vi "SerialPort.Function_Config Com Port.vi"(5 "Timeout(ms)":i32=1000, 7 "Module Name":string="Serial Port", 8 "error in":errorcluster, 9 "Port Timeout ms (3000)":u32=3000, 10 "Config":T1={"Baud Rate (115200)"=115200, "Data Bits (8)"=8, "Parity (0:none)"=enum."None", "Stop Bits (10: 1 bit)"=10, "Flow Control (0:none)"=enum."None", "Enable Term Char (T)"=TRUE, "Term Char(0xA = '\\n' = LF) "=10} {"Term Char(0xA = '\\n' = LF)" format="%.0x"; "Stop Bits (10: 1 bit)" items=["1.0"=10, "1.5"=15, "2.0"=20]; "Data Bits (8)" min=5 max=8 step=1}, 11 "Q In":refnum<queue>) -> (0 "error out":errorcluster)   [LabVIEW 2018]
uses:
  <vilib>/KATE/Queues/Q.Element.ctl
  Controls/SeroalPort.Config Settings.ctl
  <vilib>/KATE/Queues/Queue Utils.lvlib
panel:
  # "Serial Port Config"
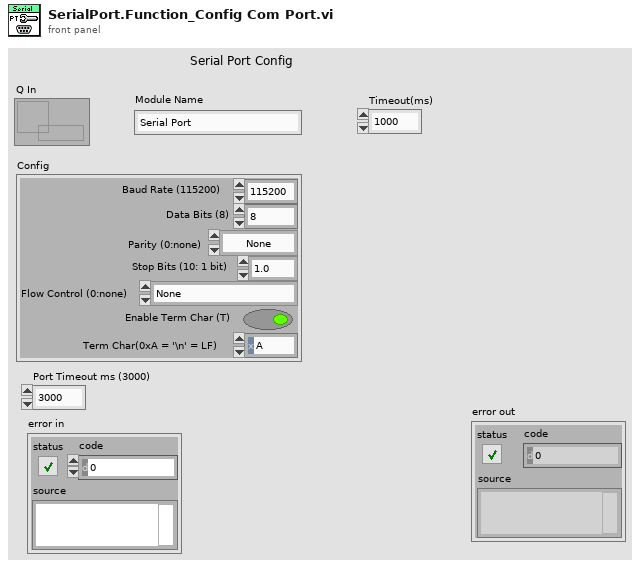
[diagram p1: front panel]
types:
  T1 = typedef "SeroalPort.Config Settings.ctl" = cluster{"Baud Rate (115200)":u32, "Data Bits (8)":u16, "Parity (0:none)":enum16{"None", "Odd", "Even", "Mark", "Space"}, "Stop Bits (10: 1 bit)":u16, "Flow Control (0:none)":enum16{"None", "XON/XOFF", "RTS/CTS", "XON/XOFF & RTS/CTS", "DTR/DSR", "XON/XOFF & DTR/DSR"}, "Enable Term Char (T)":bool, "Term Char(0xA = '\\n' = LF) ":u8}
  T2 = cluster{"Port Name":string, "Config":T1, "Port Timeout ms (3000)":u32}
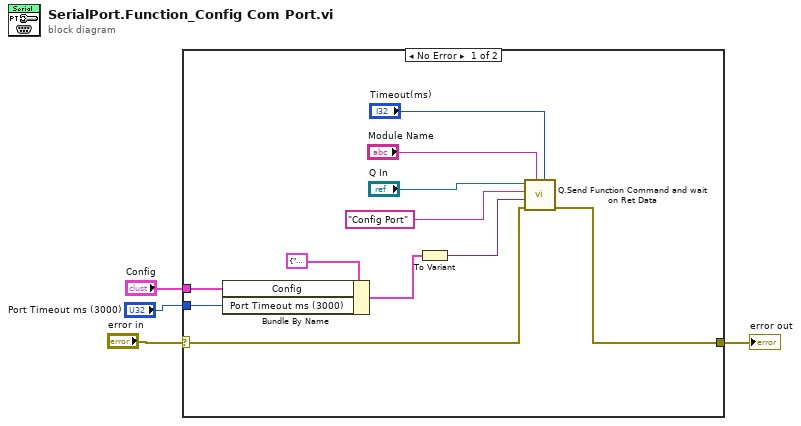
[diagram p0: block diagram]
diagram:
  n1 = case shown="No Error" "error in" {
    selector: "error in" -> [w11 w16]
    tunnel: [w10 w16] -> w3
    tunnel: "Config" -> [w6 _]
    tunnel: "Port Timeout ms (3000)" -> [w5 _]
    frame No Error {
      n2 = Bundle By Name(cluster=T2 {"Port Name"="", "Config"={"Baud Rate (115200)"=0, "Data Bits (8)"=0, "Parity (0:none)"=enum."None", "Stop Bits (10: 1 bit)"=0, "Flow Control (0:none)"=enum."None", "Enable Term Char (T)"=FALSE, "Term Char(0xA = '\\n' = LF) "=0}, "Port Timeout ms (3000)"=0} ("output cluster"), "Config"=w6, "Port Timeout ms (3000)"=w5) -> (w7:T2)
      n3 = To Variant(anything=w7) -> (Variant=w9:variant)
      n4 = call <vilib>:"Q.Send Function Command and wait on Ret Data.vi"("Timeout(ms)"="Timeout(ms)", "Q Name"="Module Name", "error in"=w11, "Data1"=w9, "Cmd"="Config Port", "Q In"="Q In") -> ("error out"=w10:errorcluster)  [unwired: 4 in, 1 out]
    }
    frame Error {
    }
  }
  "error out" <- w3
